vi "LinxI2cRead.vi"(5 "EOF":u8, 6 "Timeout (1000 ms)":u16=1000, 7 "I2C Channel":u8, 8 "Error In":errorcluster, 9 "Num Bytes":u8, 10 "Slave Address":u8, 11 "LINX Resource":T1) -> (0 "Error Out":errorcluster, 2 "Data":u8[](array[numeric]), 3 "LINX Resource":T1)   [LabVIEW 2020, in "LMH-LINX.lvlib" / "Local IO.lvlib"]
uses:
  Local IO.lvlib
  Type Defs/LINX Ref.ctl
  Type Defs/Platform.ctl
  Type Defs/Interface.ctl
  Device/Type Defs/LINX Device Config.ctl
  Device/Type Defs/TCP Config.ctl
  Device/Type Defs/Channels.ctl
  <vilib>/MakerHub/LINX/Resources/liblinxdevice.dll
  LMH-LINX.lvlib
  Device/Device.lvlib
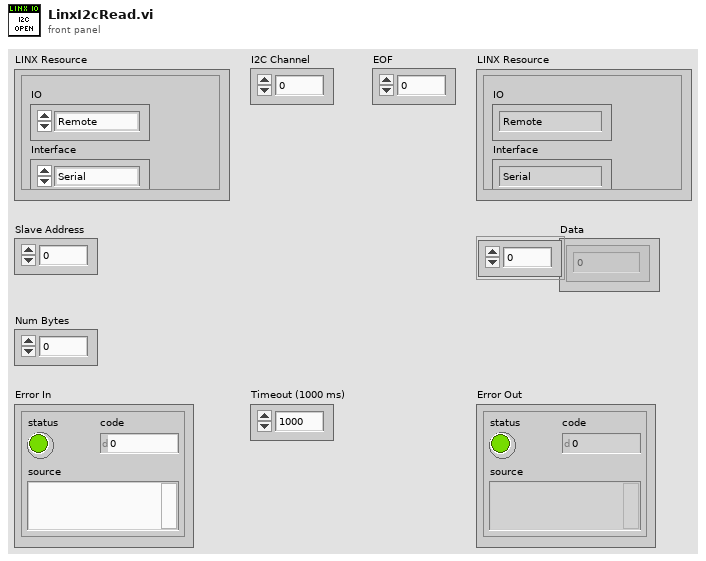
[diagram p1: front panel]
types:
  T1 = typedef "LMH-LINX.lvlib/LINX Ref.ctl" = cluster{"IO":T2, "Interface":T3, "LINX Device Config":T4}
  T2 = typedef "LMH-LINX.lvlib/Platform.ctl" = enum16{"Remote", "Local"}
  T3 = typedef "LMH-LINX.lvlib/Interface.ctl" = enum16{"Serial", "TCP"}
  T4 = typedef "LMH-LINX.lvlib/Device.lvlib/LINX Device Config.ctl" = cluster{"Interface":T3, "COM Port":refnum<visa-resource-name>, "TCP Configuration":T5, "Device Family":u8, "Device ID":u8, "Device Name":string, "TCP Ref":refnum<k5>, "Channels":T6}
  T5 = typedef "LMH-LINX.lvlib/Device.lvlib/TCP Config.ctl" = cluster{"IP Address":string, "Port":u16}
  T6 = typedef "LMH-LINX.lvlib/Channels.ctl" = cluster{"DI":u8[], "DO":u8[], "AI":u8[], "AO":u8[], "PWM":u8[], "QE":u8[], "UART":u8[], "I2C 2":u8[], "SPI":u8[], "CAN":u8[], "Servo":u8[], "AI Ref (V)":dbl, "AI Resolution (Bits)":u8, "AO Ref (V)":dbl, "AO Resolution (Bits)":u8}
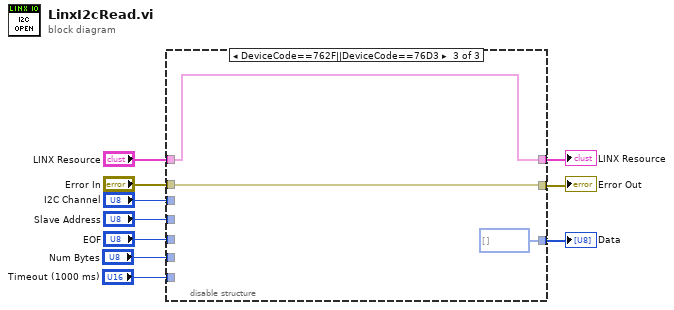
[diagram p0: block diagram]
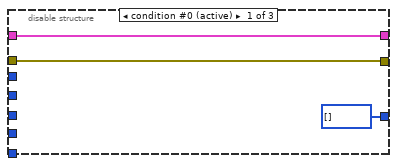
[diagram p2: hidden frame]
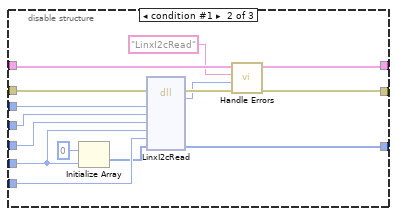
[diagram p3: hidden frame]
diagram:
  n1 = disable-structure shown="DeviceCode==762F||DeviceCode==76D3" {
    disable-tunnel: "LINX Resource" -> [w13 w27 w31]
    disable-tunnel: "Error In" -> [w12 w28 w30]
    disable-tunnel: [w12 w25 w30] -> w8
    disable-tunnel: [w13 w26 w31] -> w7
    disable-tunnel: "I2C Channel" -> [_ w21 _]
    disable-tunnel: "Slave Address" -> [_ w20 _]
    disable-tunnel: "EOF" -> [_ w19 _]
    disable-tunnel: "Timeout (1000 ms)" -> [_ w18 _]
    disable-tunnel: "Num Bytes" -> [_ w15 _]
    disable-tunnel: [u8[] [] ("Data") w14 u8[] [] ("Data")] -> w1
    frame condition #0 (active) {
    }
    frame condition #1 {
      n2 = Initialize Array(u8 0 ("dimension size"), w15) -> (w16:u8[])
      n3 = dll-call lib="C:/Program Files (x86)/National Instruments/LabVIEW 2020/vi.lib/MakerHub/LINX/Resources/liblinxdevice.*" fn="LinxI2cRead"(error in=w28, "channel"=w21, "slaveAddress"=w20, "eofConfig"=w19, "numBytes"=w15, "timeout"=w18, "recBuffer"=w16) -> (error out=w24:errorcluster, "LinxStatus"=w23:i32, "recBuffer"=w14:u8[])  [unwired: 7 in, 1 out]
      n4 = call <vilib>:"Handle Errors.vi"("Error In"=w24, "LinxStatus"=w23, "Function Name"="LinxI2cRead", "LINX Resource"=w27) -> ("Error Out"=w25:errorcluster, "LINX Resource"=w26:T1)  [unwired: 6 in]
    }
    frame condition #2 {
    }
  }
  "Error Out" <- w8
  "LINX Resource" <- w7
  "Data" <- w1
